vi "Change Wheel Type.vi"(8 "error in (no error)":errorcluster, 10 "wheel type":string, 11 "wheel in":refnum<class "NI_Robotics_Wheel.lvclass">) -> (0 "error out":errorcluster, 1 "changed?":bool, 3 "wheel out":refnum<class "NI_Robotics_Wheel.lvclass">)   [LabVIEW 2017, in "NI_Robotics_Configure Steering Frame.lvlib"]
uses:
  <vilib>/robotics/Dialog/Configure Steering Frame/NI_Robotics_Configure Steering Frame.lvlib
  <vilib>/robotics/Steering/Wheel/NI_Robotics_Wheel.lvclass
  <vilib>/robotics/Steering/Wheel/NI_Robotics_Wheel.lvclass/NI_Robotics_Wheel.ctl
  <vilib>/robotics/Steering/Steering Wheel/Steering Wheel Parameters.ctl
  <vilib>/robotics/Steering/Steering Wheel/Steering Angle Range.ctl
  <vilib>/robotics/Steering/Caster Wheel/Caster Wheel Parameters.ctl
  <vilib>/robotics/Steering/Mecanum Wheel/Roller Orientation.ctl
  <vilib>/robotics/Steering/Wheel/Get Motor Communication.vi
  <vilib>/robotics/Steering/Wheel/Get Wheel Parameters.vi
  <vilib>/robotics/Steering/Fixed Wheel/NI_Robotics_Fixed Wheel.lvclass
  c:/Program Files (x86)/National Instruments/LabVIEW 2017/vi.lib/robotics/Steering/Wheel/NI_Robotics_Wheel.lvclass
  <vilib>/robotics/Steering/Steering Wheel/NI_Robotics_Steering Wheel.lvclass
  <vilib>/robotics/Steering/Caster Wheel/NI_Robotics_Caster Wheel.lvclass
  <vilib>/robotics/Steering/Mecanum Wheel/NI_Robotics_Mecanum Wheel.lvclass
  <vilib>/robotics/Steering/Omnidirectional Wheel/NI_Robotics_Omnidirectional Wheel.lvclass
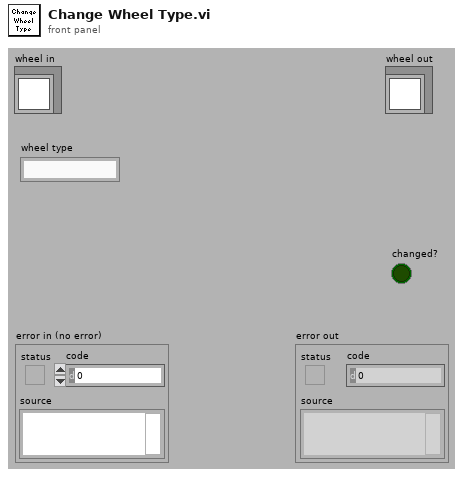
[diagram p1: front panel]
types:
  T1 = typedef "NI_Robotics_Steering Wheel.lvclass/Steering Wheel Parameters.ctl" = cluster{"steering gear ratio":dbl, "motor angle offset (rad)":dbl, "steering angle range":T2}
  T2 = typedef "NI_Robotics_Steering Wheel.lvclass/Steering Angle Range.ctl" = cluster{"min steering angle (rad)":dbl, "max steering angle (rad)":dbl}
  T3 = typedef "NI_Robotics_Caster Wheel.lvclass/Caster Wheel Parameters.ctl" = cluster{"forward offset":dbl, "caster gear ratio":dbl}
  T4 = typedef "NI_Robotics_Wheel.lvclass/Wheel Parameters.ctl" = cluster{"wheel radius":dbl, "gear ratio":dbl, "forward rotation direction":T5}
  T5 = typedef "NI_Robotics_Wheel.lvclass/Rotation Direction.ctl" = u16
  T6 = typedef "NI_Robotics_Mecanum Wheel.lvclass/Roller Orientation.ctl" = u16
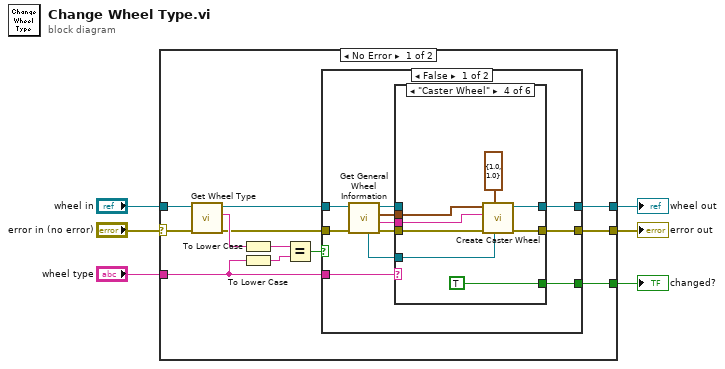
[diagram p0: block diagram]
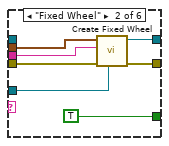
[diagram p3: hidden frame]
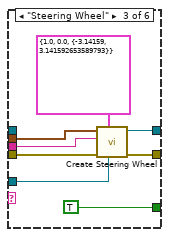
[diagram p4: hidden frame]
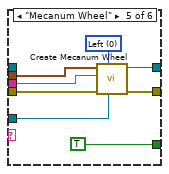
[diagram p5: hidden frame]
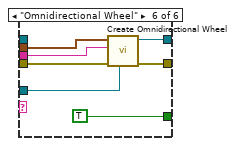
[diagram p6: hidden frame]
diagram:
  n1 = case shown="No Error" "error in (no error)" {
    selector: "error in (no error)" -> [w17 w72]
    tunnel: "wheel in" -> [w18 w73]
    tunnel: [w9 w73] -> w4
    tunnel: [w8 w72] -> w3
    tunnel: "wheel type" -> [w10 _]
    tunnel: [w7 _] -> w1
    frame No Error {
      n2 = call-dynamic "Get Wheel Type.vi"("error in (no error)"=w17, "wheel in"=w18) -> ("error out"=w11:errorcluster, "wheel type"=w15:string, "wheel out"=w12:refnum<class "NI_Robotics_Wheel.lvclass">)  [unwired: 7 in]
      n3 = To Lower Case(string=w15) -> (all lower case string=w16:string)
      n4 = To Lower Case(string=w10) -> (all lower case string=w14:string)
      n5 = Equal?(x=w16, y=w14) -> (x = y?=w13:bool)
      n6 = case shown="False" w13 {
        tunnel: w12 -> [w29 w71]
        tunnel: w11 -> [w28 w70]
        tunnel: w10 -> [w25 _]
        tunnel: [w22 w71] -> w9
        tunnel: [w21 w70] -> w8
        tunnel: [w19 _] -> w7
        frame False {
          n7 = call <vilib>:"Get General Wheel Information.vi"("error in (no error)"=w28, "wheel in"=w29) -> ("error out"=w24:errorcluster, "wheel name"=w26:string, "wheel parameters"=w27:T4, "wheel out"=w23:refnum<class "NI_Robotics_Wheel.lvclass">, "motor communication"=w20:refnum<class "NI_Robotics_Motor Communication.lvclass">)  [unwired: 5 in]
          n8 = case shown="\"Caster Wheel\"" w25 {
            tunnel: w27 -> [_ w38 w46 w54 w62 w69]
            tunnel: w26 -> [_ w37 w45 w53 w61 w68]
            tunnel: w24 -> [w30 w33 w41 w49 w57 w64]
            tunnel: w23 -> [w31 _ _ _ _ _]
            tunnel: [w31 w35 w43 w51 w59 w66] -> w22
            tunnel: [w30 w34 w42 w50 w58 w65] -> w21
            tunnel: w20 -> [_ w36 w44 w52 w60 w67]
            tunnel: [_ TRUE TRUE TRUE TRUE TRUE] -> w19
            frame Default {
            }
            frame "Fixed Wheel" {
              n9 = call <vilib>:"Create Fixed Wheel.vi"("motor communication"=w36, "error in (no error)"=w33, "wheel name"=w37, "wheel parameters"=w38) -> ("error out"=w34:errorcluster, "fixed wheel out"=w35:refnum<class "NI_Robotics_Fixed Wheel.lvclass">)  [unwired: 6 in]
            }
            frame "Steering Wheel" {
              n10 = call <vilib>:"Create Steering Wheel.vi"("motor communication"=w44, "steering parameters"=T1 {"steering gear ratio"=1.0, "motor angle offset (rad)"=0.0, "steering angle range"={"min steering angle (rad)"=-3.14159, "max steering angle (rad)"=3.141592653589793}}, "error in (no error)"=w41, "wheel name"=w45, "wheel parameters"=w46) -> ("error out"=w42:errorcluster, "steering wheel out"=w43:refnum<class "NI_Robotics_Steering Wheel.lvclass">)  [unwired: 5 in]
            }
            frame "Caster Wheel" {
              n11 = call <vilib>:"Create Caster Wheel.vi"("motor communication"=w52, "caster parameters"=T3 {"forward offset"=1.0, "caster gear ratio"=1.0}, "error in (no error)"=w49, "wheel name"=w53, "wheel parameters"=w54) -> ("error out"=w50:errorcluster, "caster wheel out"=w51:refnum<class "NI_Robotics_Caster Wheel.lvclass">)  [unwired: 5 in]
            }
            frame "Mecanum Wheel" {
              w56 = T6 0 items=["Left", "Right"] ("roller orientation")
              n12 = call <vilib>:"Create Mecanum Wheel.vi"("motor communication"=w60, "roller orientation"=w56, "error in (no error)"=w57, "wheel name"=w61, "wheel parameters"=w62) -> ("error out"=w58:errorcluster, "mecanum wheel out"=w59:refnum<class "NI_Robotics_Mecanum Wheel.lvclass">)  [unwired: 5 in]
            }
            frame "Omnidirectional Wheel" {
              n13 = call <vilib>:"Create Omnidirectional Wheel.vi"("motor communication"=w67, "error in (no error)"=w64, "wheel name"=w68, "wheel parameters"=w69) -> ("error out"=w65:errorcluster, "omni wheel out"=w66:refnum<class "NI_Robotics_Omnidirectional Wheel.lvclass">)  [unwired: 6 in]
            }
          }
        }
        frame True {
        }
      }
    }
    frame Error {
    }
  }
  "wheel out" <- w4
  "error out" <- w3
  "changed?" <- w1
